vi "Static VI.vi"() -> ()   [LabVIEW 2012]
panel:
  out "Voltage 3":dbl
  out "Voltage 2":dbl
  out "Voltage":dbl
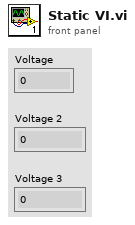
[diagram p1: front panel]
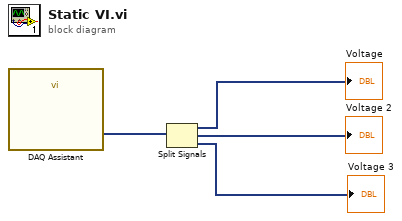
[diagram p0: block diagram]
diagram:
  n1 = call "DAQ Assistant"() -> ("data"=w4:dynamicdata)  [unwired: 17 in, 2 out]
  n2 = Split Signals(w4) -> (→"Voltage":dynamicdata, →"Voltage 2":dynamicdata, →"Voltage 3":dynamicdata)  [unwired: 3 in]
